vi "Read Elevator State.vi"(8 "error in (no error)":errorcluster, 11 "Current State Msg in":refnum<class "Current State Msg.lvclass">) -> (0 "error out":errorcluster, 2 "Elevator State":T1 {"Current Elevation" scale=0.0..100.0; "Current Travel Rate" scale=-1.0..1.0}, 3 "Current State Msg out":refnum<class "Current State Msg.lvclass">)   [LabVIEW 2014, in "Elevator.lvlib" / "Current State Msg.lvclass"]
uses:
  Current State Msg.lvclass
  Elevator Class/Elevator State.ctl
  Current State Msg.lvclass/Current State Msg.ctl
  Elevator Class/Elevator.lvclass
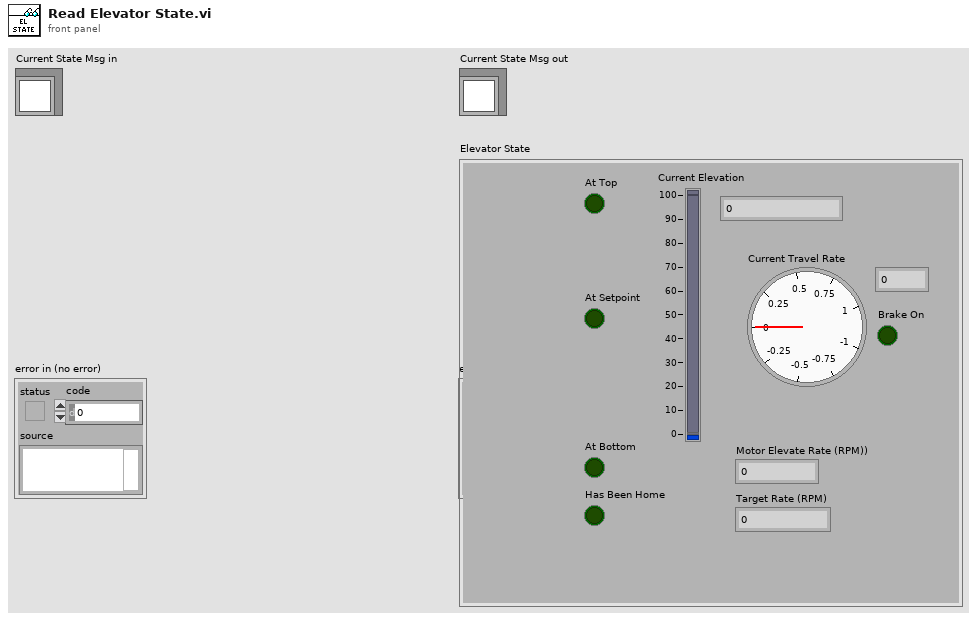
[diagram p1: front panel]
types:
  T1 = typedef "Elevator.lvlib/Elevator.lvclass/Elevator State.ctl" = cluster{"At Bottom":bool, "At Top":bool, "At Setpoint":bool, "Target Rate (RPM)":dbl, "Current Travel Rate":dbl, "Current Elevation":dbl, "Brake On":bool, "Motor Elevate Rate (RPM))":dbl, "Has Been Home":bool}
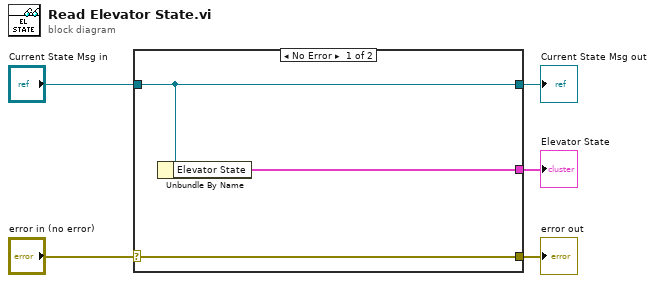
[diagram p0: block diagram]
diagram:
  n1 = case shown="No Error" "error in (no error)" {
    selector: "error in (no error)" -> [w8 w9]
    tunnel: [w8 w9] -> w4
    tunnel: [w7 w10] -> w2
    tunnel: "Current State Msg in" -> [w7 w10]
    tunnel: [w6 _] -> w1
    frame No Error {
      n2 = Unbundle By Name(w7) -> ("Elevator State"=w6:T1)
    }
    frame Error {
    }
  }
  "error out" <- w4
  "Current State Msg out" <- w2
  "Elevator State" <- w1
